vi "LIA Configure SOS.vi"(8 "error in (no error)":errorcluster, 10 "lock-in.iir config 0":T1 {"b0" format="%.17g"; "b1" format="%.17g"; "-a1" format="%.17g"; "-a2" format="%.17g"}, 11 "LIA Host Interface in":refnum<class "LIA Host Interface.lvclass">) -> (0 "error out":errorcluster, 3 "LIA Host Interface out":refnum<class "LIA Host Interface.lvclass">)   [LabVIEW 2017]
uses:
  Program Files (x86)/National Instruments/LabVIEW 2017/examples/Lock-In Amplifier/lib/interface/Interface/LIA Host Interface.lvclass
  Program Files (x86)/National Instruments/LabVIEW 2017/examples/Lock-In Amplifier/lib/interface/Interface FPGA/LIA Host Interface FPGA.lvclass
  Program Files (x86)/National Instruments/LabVIEW 2017/examples/Lock-In Amplifier/lib/host/Public/fpga type.ctl
  Program Files (x86)/National Instruments/LabVIEW 2017/examples/Lock-In Amplifier/lib/interface/Interface FPGA/Properties/FpgaSession_GET.vi
  <vilib>/Utility/error.llb/Error Cluster From Error Code.vi
  <vilib>/rvi/errors/niLvFpgaAdjustHostInterfaceError.vi
  <vilib>/rvi/interface/nirviReadWriteControl/nirviReadWriteControl.xnode
  Program Files (x86)/National Instruments/LabVIEW 2017/examples/Lock-In Amplifier/lib/host/Lock-In Amplifier Example Host.lvlib
  <vilib>/rvi/interface/Simulation/niFpgaSimulationCallBeginRW.vi
  NiFpgaLv.dll
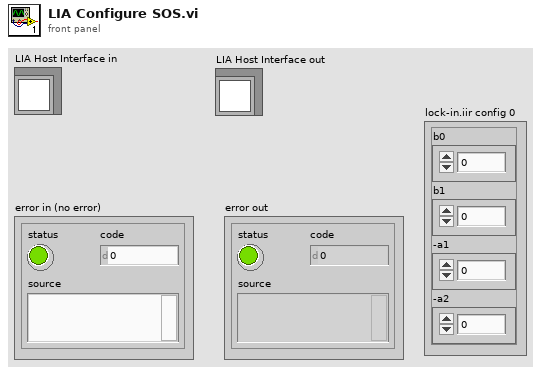
[diagram p1: front panel]
types:
  T1 = cluster{"b0":fxp<+/-,18,2>, "b1":fxp<+/-,18,2>, "-a1":fxp<+/-,18,2>, "-a2":fxp<+/-,18,2>}
  T2 = typedef "Lock-In Amplifier Example Host.lvlib/fpga type.ctl" = refnum<k20>
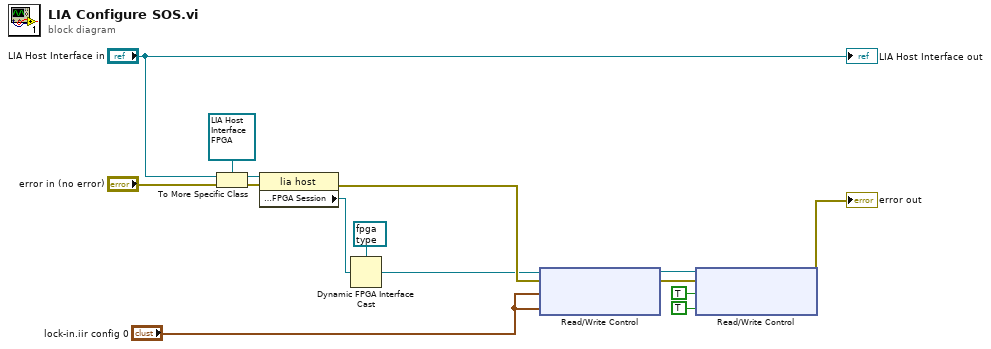
[diagram p0: block diagram]
diagram:
  n1 = To More Specific Class(target class=refnum<class "LIA Host Interface FPGA.lvclass"> refnum ("lia host"), reference="LIA Host Interface in", error in="error in (no error)") -> (specific class reference=w10:refnum<class "LIA Host Interface FPGA.lvclass">, error out=w9:errorcluster)
  n2 = property class="lia host"(reference=w10, error in=w9) -> (error out=w14:errorcluster, "Properties:FPGA Session"=w6:refnum<k20>)  [unwired: 1 out]
  n3 = Dynamic FPGA Interface Cast(Session In=T2 refnum ("fpga type"), Type=w6) -> (Session Out=w8:T2)
  n4 = xnode "Read/Write Control"("FPGA VI Reference In"=w8, "error in"=w14, "lock-in.iir config0 0"="lock-in.iir config 0", "lock-in.iir config1 0"="lock-in.iir config 0") -> ("FPGA VI Reference Out"=w11:T2, "error out"=w12:errorcluster)
  n5 = xnode "Read/Write Control"("FPGA VI Reference In"=w11, "error in"=w12, "lock-in.iir enable0 0"=TRUE ("nco.reset 0"), "lock-in.iir enable1 0"=TRUE) -> ("error out"=→"error out":errorcluster)  [unwired: 1 out]
  "LIA Host Interface out" <- "LIA Host Interface in"
